vi "PH_PowerUnit_BaseClass.evt call PU on.vi"(0 "i ref in":refnum<vi>, 1 "PowerUnit":T1, 3 "PU on":bool, 5 "error in (no error)":errorcluster) -> (14 "i ref out":refnum<vi>, 19 "error out":errorcluster)   [LabVIEW 2014, in "PH_PowerUnit_BaseClass.lvlib"]
doc: "This VI calls an event by a simple call."
uses:
  PH_PowerUnit_BaseClass.lvlib
  PH_PP_Common/PH_PP_Common.PUs.ctl
  CS_Core/CSSystem/CoreLib/CoreLib.short 2 byte array.vi
  CS_Core/CSSystem/CoreLib/CoreLib.lvlib
  CS_Core/BaseProcess/BaseProcess.lvlib
  PH_PP_Common/PH_PP_Common.lvlib
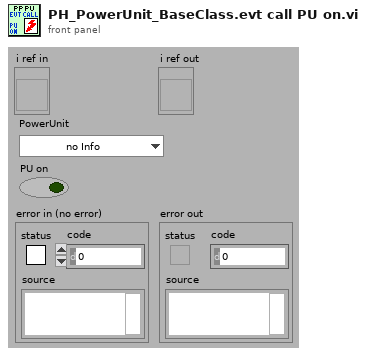
[diagram p1: front panel]
types:
  T1 = typedef "PH_PP_Common.lvlib/PH_PP_Common.PUs.ctl" = enum16{"no Info", "PA-19mm-1", "PA-19mm-2", "PA-45mm-PILC", "PA-45mm-MAIN", "MA-PU-1", "MA-PU-2", "MA-PU-3", "MA-PU-4", "MA-PU-5", "MA-PU-6", "MA-FR", "MA-PILC", "PA-45mm-DP"}
  T2 = typedef "CoreDefs.rawDataType.ctl" = i8[]
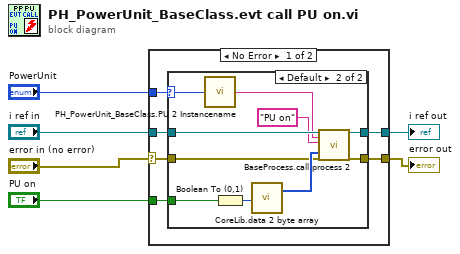
[diagram p0: block diagram]
diagram:
  n1 = case shown="No Error" "error in (no error)" {
    selector: "error in (no error)" -> [w9 w26]
    tunnel: [w12 w25] -> w2
    tunnel: [w11 w26] -> w1
    tunnel: "i ref in" -> [w10 w25]
    tunnel: "PowerUnit" -> [w8 _]
    tunnel: "PU on" -> [w7 _]
    frame No Error {
      n2 = case shown="Default" w8 {
        selector: w8 -> [_ w17]
        tunnel: [w14 w24] -> w12
        tunnel: [w13 w23] -> w11
        tunnel: w10 -> [w14 w22]
        tunnel: w9 -> [w13 w18]
        tunnel: w7 -> [_ w16]
        frame "no Info" {
        }
        frame Default {
          n3 = call "PH_PowerUnit_BaseClass.PU 2 Instancename.vi"("PU"=w17) -> ("Instance Name"=w15:string)
          n4 = Boolean To (0,1)(Boolean=w16) -> (0, 1=w20:i16)
          n5 = call-poly "CoreLib.data 2 byte array.vi"("i16"=w20) -> ("byteArray out"=w19:T2)  [unwired: 18 in]
          n6 = call "BaseProcess.call process 2.vi"("i ref in"=w22, "Object"=w15, "Selector"="PU on", "Data"=w19, "error in (no error)"=w18) -> ("i ref out"=w24:refnum<vi>, "error out"=w23:errorcluster)  [unwired: 13 in]
        }
      }
    }
    frame Error {
    }
  }
  "i ref out" <- w2
  "error out" <- w1
